vi "Wait on VIs Unloaded from Memory__ogtk.vi"(8 "error in (no error)":errorcluster, 9 "ms Polling Rate (1 ms)":u32=1, 10 "ms Timout (100ms)":u32=100, 11 "VIs to Wait on":string[](array[string])) -> (0 "error out":errorcluster, 2 "Timeout?":bool)   [LabVIEW 2018]
doc: "Waits until the VIs specified by \"VIs to Wait on\" are unloaded from memory or a timeout occurs."
panel:
  # "Wait on VIs Unloaded from Memory.vi\n\nWaits until the VIs specified by \"VIs to Wait on\" are unloaded from memory or a timeout occurs.\n\nPlease visit http://www.OpenG.org to learn about the\nOpen Source LabVIEW software movement.\n\nNOTICE -- YOU MUST LEAVE THIS NOTICE IN PLACE.  PER THE TERMS OF THE LICENSE BELOW, YOU MAY SUBLICENSE THIS SOFTWARE \nIN ANY WAY THAT DOES NOT CONFLICT WITH THIS LICENSE.\n\n### BSD License (http://www.opensource.org/licenses/bsd-license.php) Begin ###\n \nCopyright (c) 2002, Jim Kring <jim@jimkring.com>\n\nAll rights reserved.\n\nRedistribution and use in source and binary forms, with or without modification, are permitted provided that the following conditions are met:\n\n    * Redistributions of source code must retain the above copyright notice, this list of conditions and the following disclaimer.\n    * Redistributions in binary form must reproduce the above copyright notice, this list of conditions and the following disclaimer in the \n       documentation and/or other materials provided with the distribution.\n    * Neither the name of SciWare, James Kring, Inc., nor the names of its contributors may be used to endorse or promote products derived \n       from this software without specific prior written permission.\n\nTHIS SOFTWARE IS PROVIDED BY THE COPYRIGHT HOLDERS AND CONTRIBUTORS \"AS IS\" AND ANY EXPRESS OR IMPLIED WARRANTIES, \nINCLUDING, BUT NOT LIMITED TO, THE IMPLIED WARRANTIES OF MERCHANTABILITY AND FITNESS FOR A PARTICULAR PURPOSE ARE \nDISCLAIMED. IN NO EVENT SHALL THE COPYRIGHT OWNER OR CONTRIBUTORS BE LIABLE FOR ANY DIRECT, INDIRECT, INCIDENTAL,\n SPECIAL, EXEMPLARY, OR CONSEQUENTIAL DAMAGES (INCLUDING, BUT NOT LIMITED TO, PROCUREMENT OF SUBSTITUTE GOODS OR \nSERVICES; LOSS OF USE, DATA, OR PROFITS; OR BUSINESS INTERRUPTION) HOWEVER CAUSED AND ON ANY THEORY OF LIABILITY, \nWHETHER IN CONTRACT, STRICT LIABILITY, OR TORT (INCLUDING NEGLIGENCE OR OTHERWISE) ARISING IN ANY WAY OUT OF THE USE \nOF THIS SOFTWARE, EVEN IF ADVISED OF THE POSSIBILITY OF SUCH DAMAGE.\n\n### BSD License End ###"
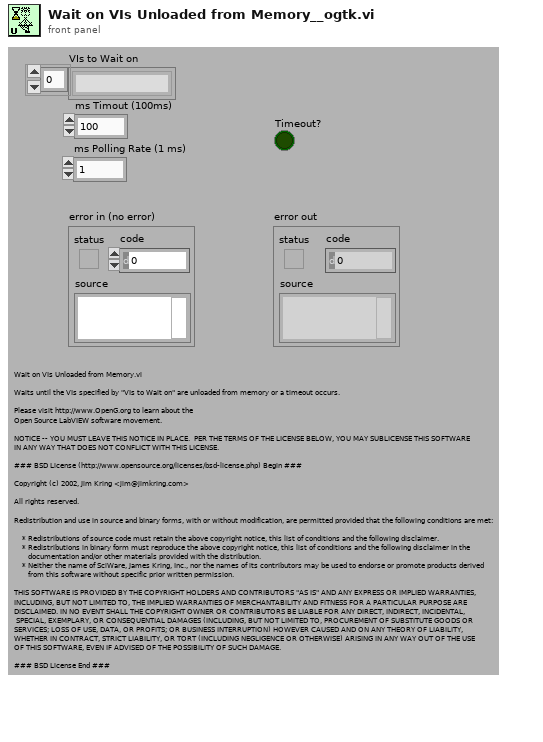
[diagram p1: front panel]
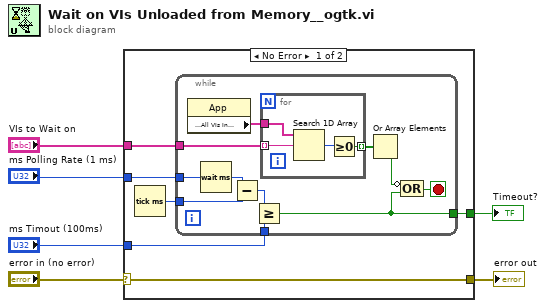
[diagram p0: block diagram]
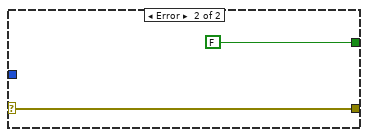
[diagram p2: hidden frame]
diagram:
  n1 = case shown="No Error" "error in (no error)" {
    selector: "error in (no error)" -> [w8 w29]
    tunnel: "VIs to Wait on" -> [w12 _]
    tunnel: "ms Timout (100ms)" -> [w10 _]
    tunnel: [w9 FALSE] -> w4
    tunnel: [w8 w29] -> w2
    tunnel: "ms Polling Rate (1 ms)" -> [w7 _]
    frame No Error {
      n2 = Tick Count (ms)() -> (millisecond timer value=w11:u32)
      n3 = while {
        tunnel: w7 -> [w13]
        tunnel: [w14] -> w9
        tunnel: w10 -> [w16]
        tunnel: w11 -> [w19]
        tunnel: w12 -> [w21]
        stop <- w15 stop-if-true
        n4 = property class="App"() -> ("Application:All VIs In Memory"=w23:string[])  [unwired: 2 in, 2 out]
        n5 = Wait (ms)(milliseconds to wait=w13) -> (millisecond timer value=w20:u32)
        n6 = Subtract(x=w20, y=w19) -> (x-y=w17:u32)
        n7 = Greater Or Equal?(x=w17, y=w16) -> (x >= y?=w14:bool)
        n8 = for {
          tunnel: w23 -> [w26]
          tunnel: w21 -> [w27] mode=indexing
          tunnel: [w24] -> w22 mode=indexing
          n9 = Search 1D Array(1D array=w26, element=w27) -> (index of element=w25:i32)  [unwired: 1 in]
          n10 = Greater Or Equal To 0?(x=w25) -> (x >= 0?=w24:bool)
        }
        n11 = Or Array Elements(Boolean array=w22) -> (logical OR=w18:bool)
        n12 = Compound Arithmetic op=OR(invert w18, w14) -> (w15:bool)
      }
    }
    frame Error {
    }
  }
  "Timeout?" <- w4
  "error out" <- w2
